vi "Motor control example.vi"() -> ()   [LabVIEW 2013]
uses:
  <vilib>/LabVIEW Interface for Arduino/LabVIEW Interface for Arduino.lvlib
panel:
  out "error out":errorcluster
  in  "Trigger/continue":bool=TRUE
  in  "Release (deg)":u8=24
  in  "Press (deg)":u8=14
  in  "stop":bool
  out "Servo 0":u8(knob) scale=0.0..180.0
  in  "Press":bool
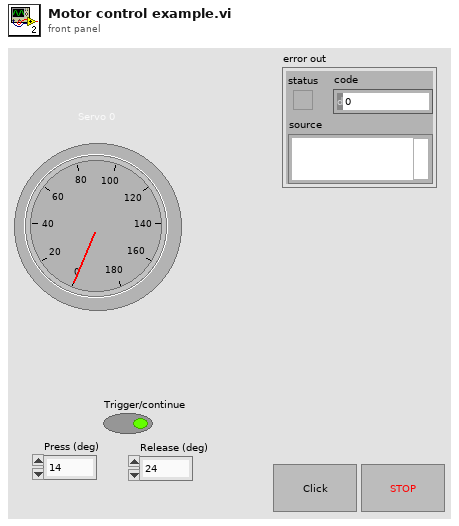
[diagram p1: front panel]
types:
  T1 = typedef "LabVIEW Interface for Arduino.lvlib/Arduino Resource.ctl" = cluster{"VISA resource":refnum<visa-resource-name>, "Board Type":T2, "Connection Type":enum8{"USB / Serial"}, "Bytes Per Packet (15)":u8}
  T2 = typedef "LabVIEW Interface for Arduino.lvlib/Board Type.ctl" = enum16{"Uno", "Dimuelanove w/Atmega 328", "Mega 2560"}
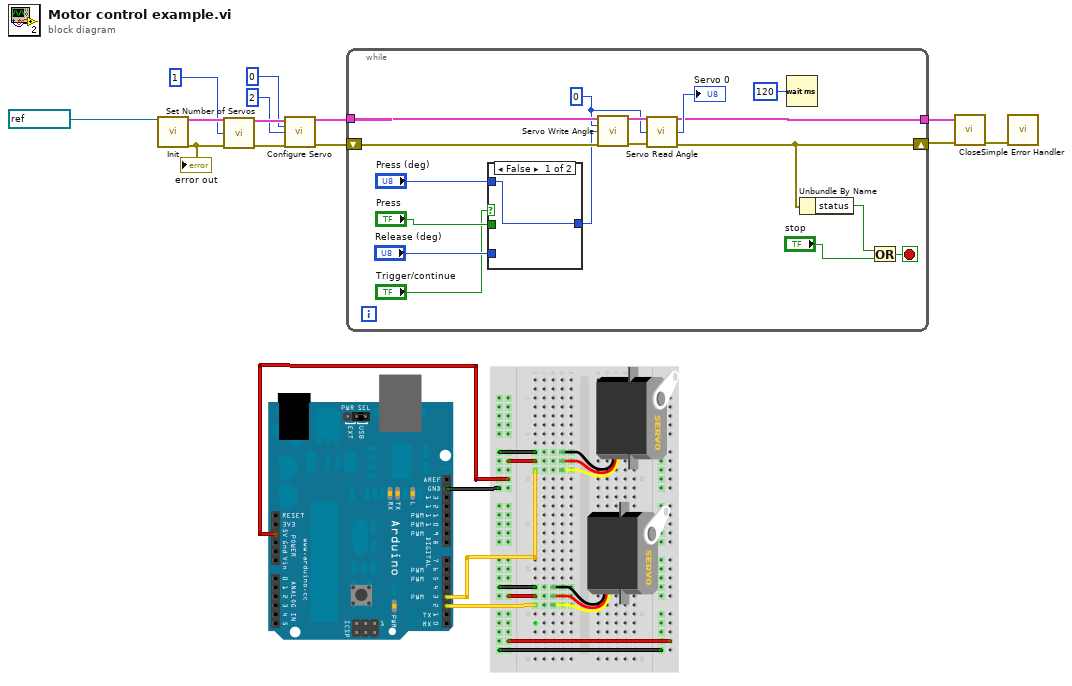
[diagram p0: block diagram]
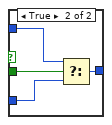
[diagram p2: hidden frame]
diagram:
  n1 = call <vilib>:"Init.vi"("VISA resource"=refnum<visa-resource-name> "COM3") -> ("Arduino Resource"=w13:T1, "error out"=w12:errorcluster)  [unwired: 17 in]
  "error out" <- w12
  n2 = call <vilib>:"Set Number of Servos.vi"("Arduino Resource"=w13, "Number Of Servos (1)"=u8 1, "error in"=w12) -> ("Arduino Resource"=w11:T1, "error out"=w10:errorcluster)  [unwired: 11 in]
  n3 = call <vilib>:"Configure Servo.vi"("Arduino Resource"=w11, "Servo Number (0)"=u8 0 ("Servo Number"), "DIO Pin (2)"=u8 2 ("Servo Number"), "error in"=w10) -> ("Arduino Resource"=w3:T1, "error out"=w2:errorcluster)  [unwired: 10 in]
  n4 = while {
    tunnel: w3 -> [w30]
    tunnel: [w22] -> w6
    shift-right: [w21] -> w7
    shift-left: w2 -> [w28]
    stop <- w26 stop-if-true
    w24 = u8 0 ("Servo Number")
    n5 = case shown="False" "Trigger/continue" {
      tunnel: "Release (deg)" -> [_ w35]
      tunnel: "Press (deg)" -> [w31 w34]
      tunnel: [w31 w33] -> w16
      tunnel: "Press" -> [_ w32]
      frame False {
      }
      frame True {
        n6 = Select(t=w34, s=w32, f=w35) -> (s? t:f=w33:u8)
      }
    }
    n7 = call <vilib>:"Servo Write Angle.vi"("Arduino Resource"=w30, "Servo Number"=w24, "Angle (Degrees)"=w16, "error in"=w28) -> ("Arduino Resource"=w29:T1, "error out"=w27:errorcluster)  [unwired: 10 in]
    n8 = call <vilib>:"Servo Read Angle.vi"("Arduino Resource"=w29, "Servo Number"=w24, "error in"=w27) -> ("Arduino Resource"=w22:T1, "Angle (Degrees)"=→"Servo 0":u8, "error out"=w21:errorcluster)  [unwired: 10 in]
    n9 = Wait (ms)(milliseconds to wait=u32 120) -> ()  [unwired: 1 out]
    n10 = Unbundle By Name(w21) -> ("status"=w25:bool)
    n11 = Or(x=w25, y="stop") -> (x .or. y?=w26:bool)
  }
  n12 = call <vilib>:"Close.vi"("Arduino Resource"=w6, "error in"=w7) -> ("error out"=w4:errorcluster)  [unwired: 13 in]
  n13 = call <vilib>:"Simple Error Handler.vi"("error in (no error)"=w4) -> ()  [unwired: 4 in, 5 out]
